vi "driveStraight.vi"(10 "Speed (ft/sec)":dbl, 11 "Distance":dbl) -> ()   [LabVIEW 2011]
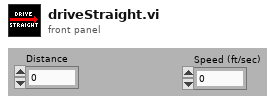
[diagram p1: front panel]
types:
  T1 = typedef "WPI_RobotDriveDevRef.ctl" = cluster{"DevStatus":errorcluster, "Motors[]":T2[], "Square Inputs":bool, "Max Output":dbl, "Isochronous":bool}
  T2 = typedef "WPI_MotorControlDeviceRef.ctl" = cluster{"DeviceStatus":errorcluster, "Type":enum16{"PWM", "CAN"}, "PWM":cluster{"Digital Module":T3, "PWM Channel":T4, "DeadBand":T5}, "CAN":cluster{"Device Number":u8, "Control Mode":T6, "Semaphore":T7, "Max Vout":dbl}, "Invert":bool, "TransformRef":T8, "InvTransformRef":T8}
  T3 = typedef "FPGA_TypedefDigitalModule.ctl" = enum16{"Digital Module 1", "Digital Module 2"}
  T4 = typedef "FPGA_DIOPWMChannel.ctl" = enum8{"PWM 1", "PWM 2", "PWM 3", "PWM 4", "PWM 5", "PWM 6", "PWM 7", "PWM 8", "PWM 9", "PWM 10", "Invalid"}
  T5 = typedef "WPI_PWMDeadband.ctl" = cluster{"Name":string, "maxPositivePwm":i32, "minPositivePwm":i32, "centerPwm":i32, "maxNegativePwm":i32, "minNegativePwm":i32, "angularRange":u16}
  T6 = typedef "WPI_CANJaguar_ControlMode.ctl" = enum8{"Percent VBus", "Current", "Speed", "Position", "Voltage"}
  T7 = typedef "Semaphore RefNum" = refnum<k1>
  T8 = typedef "WPI_PWMTransform_ConPane.ctl" = refnum<vi>
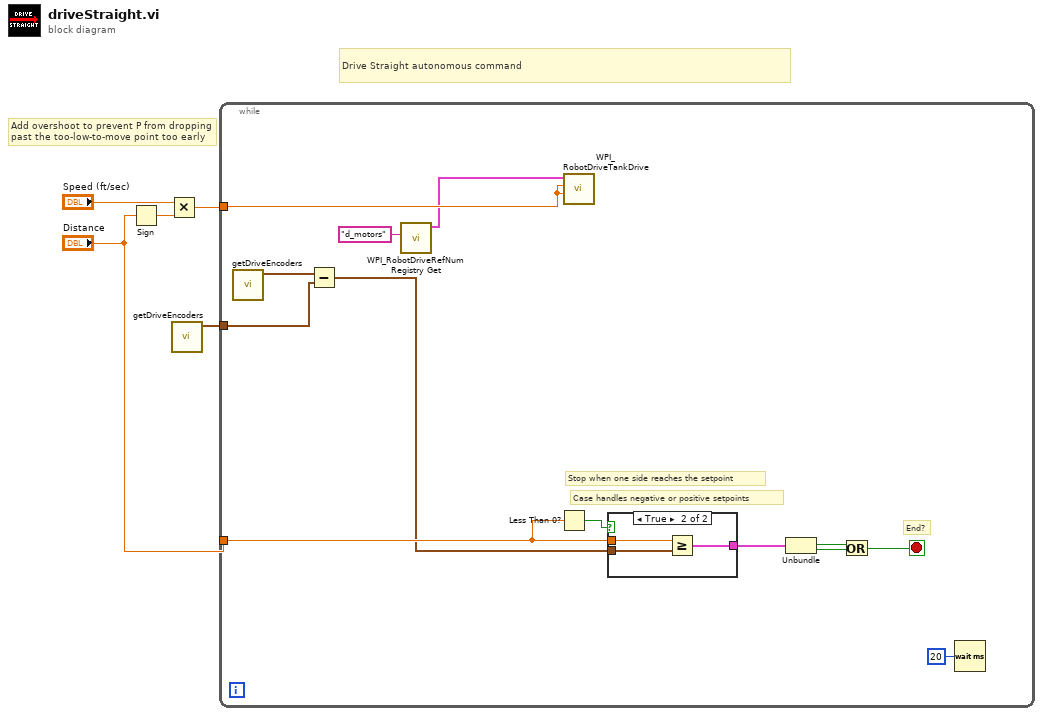
[diagram p0: block diagram]
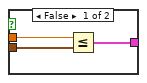
[diagram p2: hidden frame]
diagram:
  # "Drive Straight autonomous command"
  # "Add overshoot to prevent P from dropping\npast the too-low-to-move point too early"
  n1 = Sign(1:"Distance") -> (0:w2:dbl)
  n2 = Multiply(x="Speed (ft/sec)", y=w2) -> (x*y=w4:dbl)
  n3 = call "getDriveEncoders.vi"() -> ("Distance"=w5:cluster{"Left":dbl, "Right":dbl})  [unwired: 11 out]
  n4 = while {
    tunnel: w4 -> [w7]
    tunnel: w5 -> [w10]
    tunnel: "Distance" -> [w12]
    stop <- w15 stop-if-true
    # "Case handles negative or positive setpoints"
    # "End?"
    # "Stop when one side reaches the setpoint"
    n5 = call "getDriveEncoders.vi"() -> ("Distance"=w11:cluster{"Left":dbl, "Right":dbl})  [unwired: 11 out]
    n6 = Subtract(x=w11, y=w10) -> (x-y=w9:cluster{"Left":dbl, "Right":dbl})
    n7 = call <vilib>:"WPI_RobotDriveRefNum Registry Get.vi"("refnum name"="d_motors") -> ("RobotDriveDevRef"=w6:T1)  [unwired: 1 in, 9 out]
    n8 = Less Than 0?(x=w12) -> (x < 0?=w13:bool)
    n9 = call <vilib>:"WPI_RobotDriveTankDrive.vi"("Right axis value"=w7, "Left axis value"=w7, "RobotDriveDevRef"=w6) -> ()  [unwired: 1 in, 8 out]
    n10 = case shown="True" w13 {
      tunnel: w12 -> [w21 w24]
      tunnel: w9 -> [w20 w23]
      tunnel: [w19 w22] -> w18
      frame False {
        n11 = Less Or Equal?(x=w21, y=w20) -> (x <= y?=w19:cluster{"Left":bool, "Right":bool})
      }
      frame True {
        n12 = Greater Or Equal?(x=w24, y=w23) -> (x >= y?=w22:cluster{"Left":bool, "Right":bool})
      }
    }
    n13 = Unbundle(w18) -> ("Left"=w17:bool, "Right"=w16:bool)
    n14 = Or(x=w17, y=w16) -> (x .or. y?=w15:bool)
    n15 = Wait (ms)(milliseconds to wait=u32 20) -> ()  [unwired: 1 out]
  }
